vi "Get Raw Data.vi"(8 "error in (no error)":errorcluster, 11 "Red Pitaya Digitizer in":refnum<class "Red Pitaya Digitizer.lvclass">) -> (0 "error out":errorcluster, 1 "appended array":i16[][](array[numeric]), 3 "Red Pitaya Digitizer out":refnum<class "Red Pitaya Digitizer.lvclass">)   [LabVIEW 2019, in "Red Pitaya Digitizer.lvclass"]
uses:
  Red Pitaya Digitizer.lvclass
  C:/GitHub/NHMFL_Core/Libraries/Instruments/Pulse Driver/Pulse Driver.lvclass
  Red Pitaya Digitizer.lvclass/Red Pitaya Digitizer.ctl
  Instruments/Pulse Driver/Pulse Driver.lvclass/Pulse Driver.ctl
  Read RP Instrument.vi
  Instruments/Pulse Driver/Read Pretrigger samples.vi
  Instruments/Pulse Driver/Read Samples per channel.vi
  Instruments/Pulse Driver/Read Current read position.vi
  Write RP Instrument.vi
  RP Core/RP Instrument/RP Instrument.lvclass
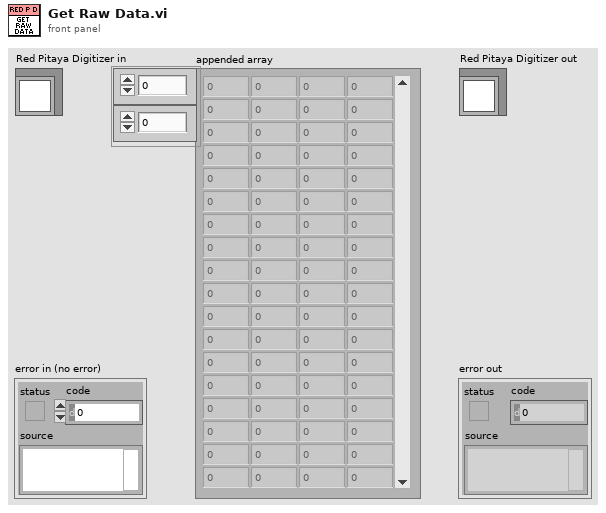
[diagram p1: front panel]
types:
  T1 = enum16{"big-endian, network order", "native, host order", "little-endian"}
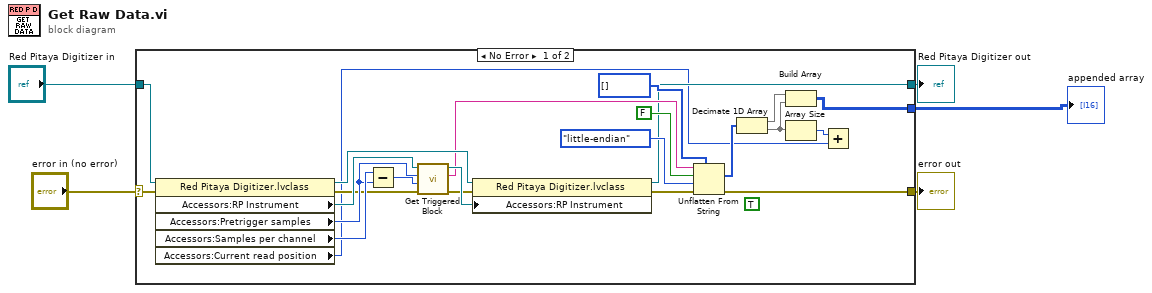
[diagram p0: block diagram]
diagram:
  n1 = case shown="No Error" "error in (no error)" {
    selector: "error in (no error)" -> [w10 w30]
    tunnel: [w8 w30] -> w4
    tunnel: [w9 w29] -> w2
    tunnel: "Red Pitaya Digitizer in" -> [w20 w29]
    tunnel: [w6 _] -> w1
    frame No Error {
      (unwired) TRUE ("Finished")
      n2 = property class="Red Pitaya Digitizer.lvclass"(reference=w20, error in=w10) -> (reference out=w28:refnum<class "Red Pitaya Digitizer.lvclass">, error out=w23:errorcluster, "Accessors:RP Instrument"=w27:refnum<class "RP Instrument.lvclass">, "Accessors:Pretrigger samples"=w25:u32, "Accessors:Samples per channel"=w26:i32, "Accessors:Current read position"=w7:i32)
      n3 = Subtract(x=w26, y=w25) -> (x-y=w24:u32)
      n4 = call-dynamic "Get Triggered Block.vi"("error in (no error)"=w23, "Post-trigger points"=w24, "Pre-trigger points"=w25, "RP Instrument in"=w27) -> ("error out"=w21:errorcluster, "Data out"=w12:string, "RP Instrument out"=w22:refnum<class "RP Instrument.lvclass">)  [unwired: 5 in]
      n5 = property class="Red Pitaya Digitizer.lvclass"(reference=w28, error in=w21, "Accessors:RP Instrument"=w22) -> (reference out=w9:refnum<class "Red Pitaya Digitizer.lvclass">, error out=w11:errorcluster)
      n6 = Unflatten From String(type=i16[] [], binary string=w12, data includes array or string size? (T)=FALSE, byte order (0:big-endian, network order)=T1."little-endian", error in (no error)=w11) -> (value=w14:i16[], error out=w8:errorcluster)  [unwired: 1 out]
      n7 = Decimate 1D Array(w14) -> (w13:i16[], w18:i16[])
      n8 = Build Array(w13, w18) -> (w6:i16[][])
      n9 = Array Size(array=w18) -> (size(s)=w19:i32)
      n10 = Add(x=w19, y=w7) -> ()  [unwired: 1 out]
    }
    frame Error {
    }
  }
  "error out" <- w4
  "Red Pitaya Digitizer out" <- w2
  "appended array" <- w1
